vi "resolution_to_timebase.vi"(11 "Resolution (s)":dbl) -> (3 "15 bit Timebase":dbl)   [LabVIEW 2016]
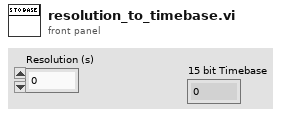
[diagram p1: front panel]
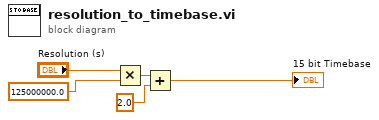
[diagram p0: block diagram]
diagram:
  n1 = Multiply(x="Resolution (s)", y=125000000.0) -> (x*y=w3:dbl)
  n2 = Add(x=w3, y=2.0) -> (x+y=→"15 bit Timebase":dbl)
